vi "Popup - Add Sensor.vi"() -> (2 "Output Sensor":T1, 3 "Cancelled?":bool)   [LabVIEW 2020]
panel:
  in  "Low Pressure?":bool
  in  "Cancel Button":bool
  in  "Add Button":bool
  in  "Serial No.":string
  in  "Description":string
  in  "ID":string
  in  "Type":string
  # "ADD SENSOR"
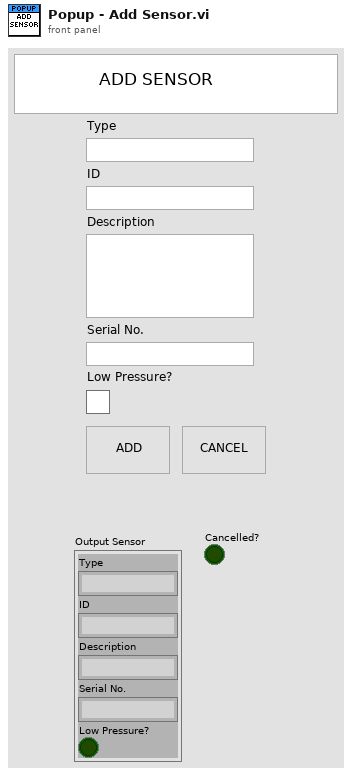
[diagram p1: front panel]
types:
  T1 = cluster{"Type":string, "ID":string, "Description":string, "Serial No.":string, "Low Pressure?":bool}
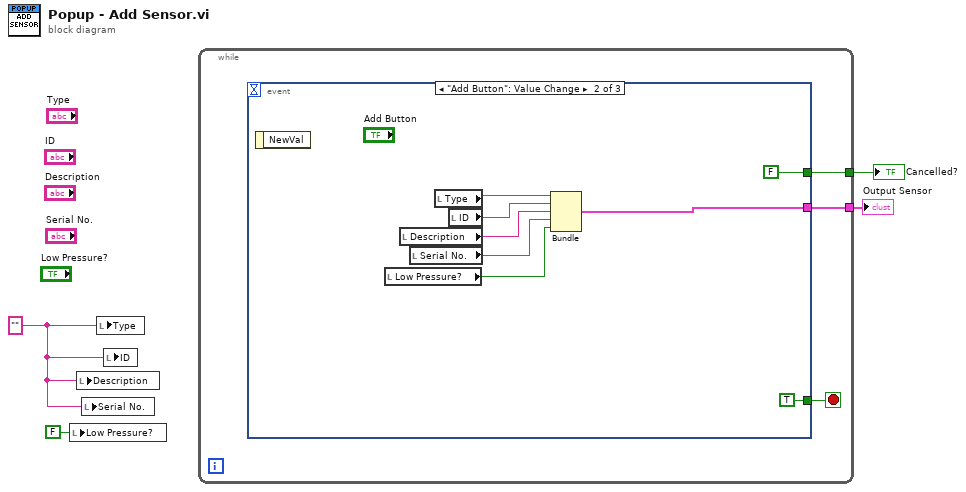
[diagram p0: block diagram]
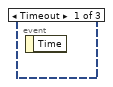
[diagram p2: hidden frame]
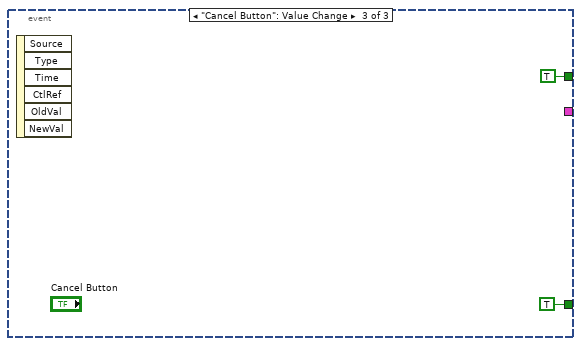
[diagram p3: hidden frame]
diagram:
  w2 = "" ("Type")
  n1 = local write "Low Pressure?"(FALSE ("Low Pressure?")) -> ()
  n2 = local write "Description"(w2) -> ()
  n3 = local write "Serial No."(w2) -> ()
  n4 = local write "Type"(w2) -> ()
  n5 = local write "ID"(w2) -> ()
  n6 = while {
    tunnel: [w7] -> w3
    tunnel: [w6] -> w4
    stop <- w5 stop-if-true
    n7 = event shown="[1] \"Add Button\": Value Change" {
      selector: _ -> [_ _ _]
      dyn-events: _ -> [_ _ _]
      timeout: _ -> [_ _ _]
      tunnel: [_ w11 _] -> w7
      tunnel: [_ FALSE TRUE] -> w6
      tunnel: [_ TRUE TRUE] -> w5
      event Timeout {
        n8 = event-data() -> ()  [unwired: 1 in, 1 out]
      }
      event "Add Button": Value Change {
        n9 = event-data() -> ()  [unwired: 1 in, 1 out]
        n10 = local read "Low Pressure?"() -> (w8:bool)
        n11 = local read "Description"() -> (w13:string)
        n12 = local read "Serial No."() -> (w12:string)
        n13 = local read "Type"() -> (w15:string)
        n14 = local read "ID"() -> (w14:string)
        n15 = Bundle("Type"=w15, "ID"=w14, "Description"=w13, "Serial No."=w12, "Low Pressure?"=w8) -> (w11:T1)  [unwired: 1 in]
      }
      event "Cancel Button": Value Change {
        n16 = event-data() -> ()  [unwired: 1 in, 6 out]
      }
    }
  }
  "Cancelled?" <- w4
  "Output Sensor" <- w3
